vi "E727_Sample_Application_HenryEdit.vi"() -> ()   [LabVIEW 2022 SP3]
doc: "This VI demonstrates how to initialize an E-727 system, how to move one connected axis and how to query for the position value of this axis. \nIn this example the E-727 is connected through COM port 1 with baudrate 115200. The VI runs E727_Configuration_Setup.vi with these specified settings, moves the first connected axis relative to its current position and reads the position of this axis. The diagram shows how to combine the driver VIs for these tasks. \nWarning: Before running this VI, modify the \"Interface\" and \"RS232 settings\" (or TCP/IP settings or USB settings ) to reflect your configuration. The predefined settings provided with the VI probably do not match your system."
panel:
  in  "x":dbl[](array[numeric])
  out "number":u32
  out "Array":dbl[](array[numeric])
  out "Initial position":dbl[](array[numeric]) format="%.6f"
  in  "stop":bool
  in  "error in":errorcluster
  out "Running":bool caption="Configuration_Setup.vi is running"
  out "error out":errorcluster
  out "Final position":dbl[](array[numeric]) format="%.6f"
  out "Conn. Axis":string[](array[string])
  out "Identification":string
  # "This VI demonstrates how to initialize an E-727 system, how to move one axis and how to query for the position value of this axis. \nThe VI runs E727_Configuration_Setup.vi with specified settings, moves the first axis relative to its current position and reads the\nposition of this axis. The diagram shows how to combine the driver VIs for these tasks. \n\nWarning: Before running this VI, modify the interface settings on the block diagram to reflect your configuration. The predefined \n                 settings provided with the VI probably do not match your system."
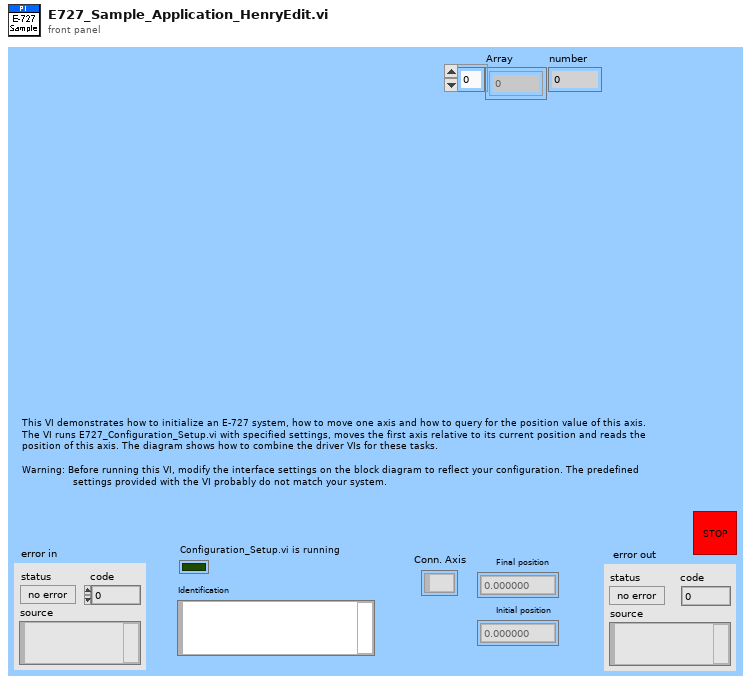
[diagram p1: front panel]
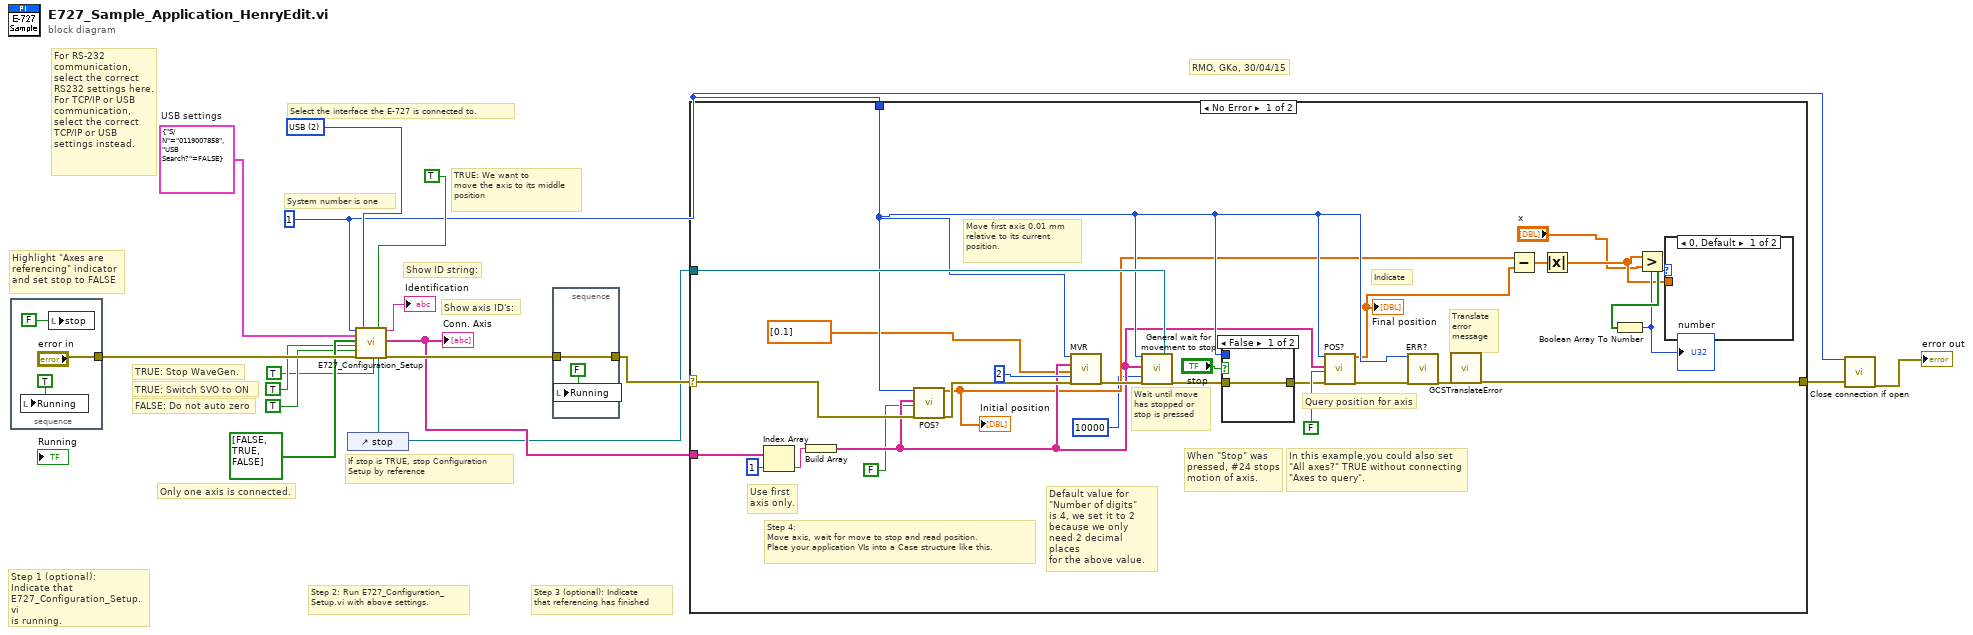
[diagram p0: block diagram]
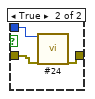
[diagram p2: hidden frame]
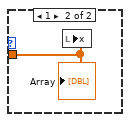
[diagram p3: hidden frame]
diagram:
  w1 = cluster{"S/N":string, "USB Search?":bool} {"S/N"="0119007858", "USB Search?"=FALSE}  # USB settings
  w8 = u16 2 items=["RS232", "TCP/IP", "USB"] ("Interface")
  w3 = 1 ("System no.")
  # "RMO, GKo, 30/04/15"
  # "Only one axis is connected."
  # "TRUE: We want to\nmove the axis to its middle\nposition"
  # "FALSE: Do not auto zero"
  # "TRUE: Switch SVO to ON"
  # "If stop is TRUE, stop Configuration\nSetup by reference"
  # "For RS-232 \ncommunication,\nselect the correct\nRS232 settings here.\nFor TCP/IP or USB \ncommunication, \nselect the correct \nTCP/IP or USB\nsettings instead."
  # "Select the interface the E-727 is connected to."
  # "Step 3 (optional): Indicate\nthat referencing has finished"
  # "Step 2: Run E727_Configuration_\nSetup.vi with above settings."
  # "Step 1 (optional): \nIndicate that\nE727_Configuration_Setup.vi\nis running."
  # "Highlight \"Axes are\nreferencing\" indicator\nand set stop to FALSE"
  # "Show axis ID's:"
  # "Show ID string:"
  # "TRUE: Stop WaveGen."
  # "System number is one"
  n1 = stacked-sequence {
    tunnel: ["error in"] -> w14
    frame #0 {
      n2 = local write "Running"(TRUE ("Running")) -> ()
      n3 = local write "stop"(FALSE ("stop")) -> ()
    }
  }
  n4 = control-ref of="stop"() -> (w2:refnum<vi>)
  n5 = call "E727_Configuration_Setup.vi"("System no."=w3, "USB settings"=w1, "Are stages connected?"=bool[] [FALSE, TRUE, FALSE], "Change servo status to ON?"=TRUE ("Use dialog to define\nconnected stages?"), "Perform autozero?"=TRUE ("Use dialog to define\nconnected stages?"), "error in"=w14, "Interface"=w8, "Stop wave generator\noutput (if any)"=TRUE ("All axes?"), "Move to middle?"=TRUE, "Stop refnum"=w2) -> ("Identification"=→"Identification":string, "All conn. axes"=w5:string[], "error out"=w13:errorcluster)  [unwired: 4 in, 3 out]
  "Conn. Axis" <- w5
  n6 = stacked-sequence {
    tunnel: w13 -> [w21]
    tunnel: [w21] -> w4
    frame #0 {
      n7 = local write "Running"(FALSE ("Running")) -> ()
    }
  }
  n8 = case shown="No Error" w4 {
    selector: w4 -> [w46 w54]
    tunnel: w5 -> [w47 _]
    tunnel: w3 -> [w45 _]
    tunnel: w2 -> [w48 _]
    tunnel: [w44 w54] -> w15
    frame No Error {
      # "Step 4: \nMove axis, wait for move to stop and read position.\nPlace your application VIs into a Case structure like this."
      # "Use first\naxis only."
      # "When \"Stop\" was \npressed, #24 stops\nmotion of axis."
      # "Translate\nerror \nmessage"
      # "Wait until move\nhas stopped or\nstop is pressed"
      # "Indicate"
      # "Default value for\n\"Number of digits\"\nis 4, we set it to 2\nbecause we only\nneed 2 decimal places\nfor the above value."
      # "Move first axis 0.01 mm\nrelative to its current\nposition."
      # "In this example,you could also set \n\"All axes?\" TRUE without connecting\n\"Axes to query\"."
      # "Query position for axis"
      n9 = Index Array(array=w47, index=1) -> (element=w34:string)
      n10 = Build Array(w34) -> (w32:string[])
      n11 = call "POS?.vi"("System no."=w45, "Axes to query"=w32, "All axes?"=FALSE, "error in"=w46) -> ("Position"=w30:dbl[], "error out"=w33:errorcluster)  [unwired: 1 in, 13 out]
      "Initial position" <- w30
      n12 = call "MVR.vi"("System no."=w45, "Axes to move"=w32, "Position values"=dbl[] [0.1], "No.of digits"=i16 2, "error in"=w33) -> ("error out"=w41:errorcluster)  [unwired: 14 out]
      n13 = call "General wait for movement to stop.vi"("System no."=w45, "Axes to wait for"=w32, "Additional wait time, ms"=u32 10000, "error in"=w41, "Stop refnum"=w48) -> ("error out"=w40:errorcluster)  [unwired: 3 in, 11 out]
      n14 = case shown="False" "stop" {
        tunnel: w40 -> [w49 w52]
        tunnel: [w49 w51] -> w39
        tunnel: w45 -> [_ w50]
        frame False {
        }
        frame True {
          n15 = call "#24.vi"("System no."=w50, "error in"=w52) -> ("error out"=w51:errorcluster)  [unwired: 17 out]
        }
      }
      n16 = call "POS?.vi"("System no."=w45, "Axes to query"=w32, "All axes?"=FALSE, "error in"=w39) -> ("Position"=w29:dbl[], "error out"=w37:errorcluster)  [unwired: 1 in, 13 out]
      "Final position" <- w29
      n17 = call "ERR?.vi"("System no."=w45, "error in"=w37) -> ("error out"=w36:errorcluster)  [unwired: 17 out]
      n18 = call "GCSTranslateError.vi"("error in"=w36) -> ("error out"=w44:errorcluster)  [unwired: 18 out]
      n19 = Subtract(x=w30, y=w29) -> (x-y=w26:dbl[])
      n20 = Absolute Value(x=w26) -> (abs(x)=w25:dbl[])
      n21 = Greater?(x=w25, y="x") -> (0:w28:bool[])
      n22 = Boolean Array To Number(Boolean array=w28) -> (number=w27:u32)
      "number" <- w27
      n23 = case shown="0, Default" w27 {
        tunnel: w25 -> [_ w53]
        frame 0, Default {
        }
        frame 1 {
          n24 = local write "x"(w53) -> ()
          "Array" <- w53
        }
      }
    }
    frame Error {
      # "Error during initialization"
    }
  }
  n25 = call "Close connection if open.vi"("System no."=w3, "error in"=w15) -> ("error out"=→"error out":errorcluster)  [unwired: 1 in, 16 out]
